vi "Format Fixed Header.vi"(8 "RETAIN":bool, 9 "QoS":T1, 10 "DUP":bool, 11 "Control Packet Type":T2) -> (3 "Fixed Header":u8 format="%08b")   [LabVIEW 2013]
uses:
  Control Packet Type -- enum.ctl
  QualityOfService -- enum.ctl
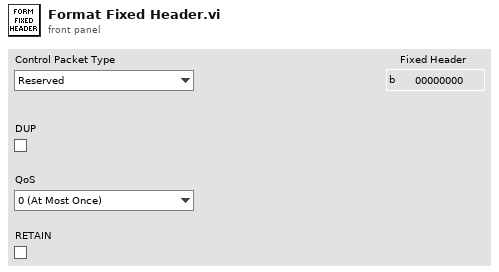
[diagram p1: front panel]
types:
  T1 = typedef "QualityOfService -- enum.ctl" = enum16{"0 (At Most Once)", "1 (At Least Once)", "2 (Exactly Once)"}
  T2 = typedef "Control Packet Type -- enum.ctl" = enum16{"Reserved", "CONNECT", "CONNACK", "PUBLISH", "PUBACK", "PUBREC", "PUBREL", "PUBCOMP", "SUBSCRIBE", "SUBACK", "UNSUBSCRIBE", "UNSUBACK", "PINGREQ", "PINGRESP", "DISCONNECT", "Reserved(15)"}
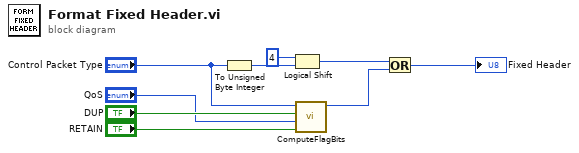
[diagram p0: block diagram]
diagram:
  n1 = To Unsigned Byte Integer(number="Control Packet Type") -> (unsigned 8bit integer=w3:u8)
  n2 = Logical Shift(y=i16 4, x=w3) -> (x << y=w1:u8)
  n3 = call "ComputeFlagBits.vi"("RETAIN"="RETAIN", "QoS"="QoS", "DUP"="DUP", "Control Packet Type"="Control Packet Type") -> ("Flag Bits"=w2:u8)  [unwired: 7 in]
  n4 = Or(x=w1, y=w2) -> (x .or. y?=→"Fixed Header":u8)
